vi "getADC.vi"(8 "error in (no error)":errorcluster, 10 "ILC In":refnum<class "ILC.lvclass">, 11 "IILCADC in":refnum<class "IILCADC.lvclass">) -> (0 "error out":errorcluster, 1 "ADC Value":dbl[unit], 2 "ILC Out":refnum<class "ILC.lvclass">, 3 "IILCADC out":refnum<class "IILCADC.lvclass">)   [LabVIEW 2015, in "IILCADC.lvclass"]
uses:
  IILCADC.lvclass
  <userlib>/Common/ILC/ILC/ILC.lvclass
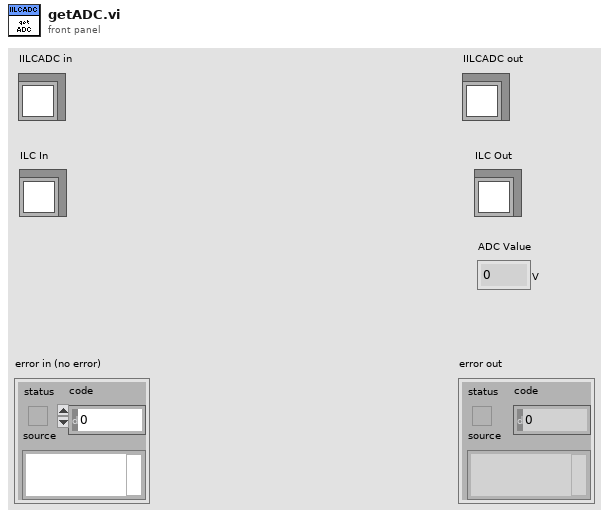
[diagram p1: front panel]
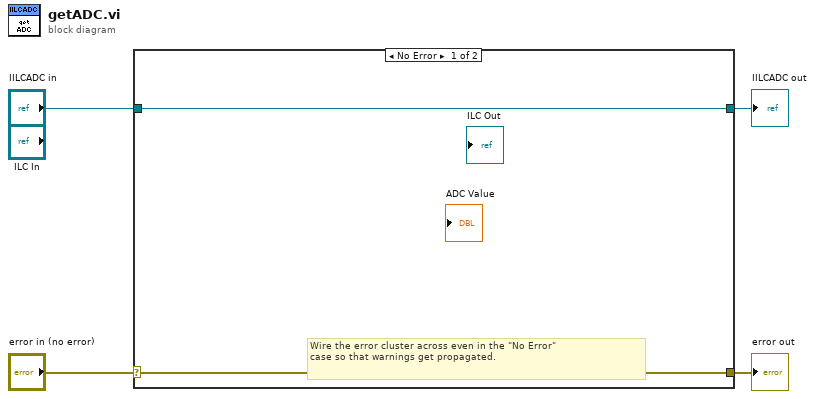
[diagram p0: block diagram]
diagram:
  n1 = case shown="No Error" "error in (no error)" {
    selector: "error in (no error)" -> [w5 w8]
    tunnel: [w5 w8] -> w3
    tunnel: [w6 w7] -> w1
    tunnel: "IILCADC in" -> [w6 w7]
    frame No Error {
      # "Wire the error cluster across even in the \"No Error\"\ncase so that warnings get propagated."
    }
    frame Error {
    }
  }
  "error out" <- w3
  "IILCADC out" <- w1
